vi "TC560-Write Command Data.vi"(8 "error in":errorcluster, 11 "Configuration":T1={"Connection Setting"={"VISA Resource Name"="", "Baud Rate"=9600, "Parity"=0, "Flow Control"=0}, "Wait For Read"=0} {"Connection Setting"."Flow Control" items=["None", "XON/XOFF", "RTS/CTS", "XON/XOFF & RTS/CTS", "DTR/DSR", "XON/XOFF & DTR/DSR"]; "Connection Setting"."Parity" items=["None", "Odd", "Even", "Mark", "Space"]; "Connection Setting"."Baud Rate" items=["2400"=2400, "4800"=4800, "9600"=9600]}) -> (0 "error out":errorcluster)   [LabVIEW 2018]
uses:
  Data Def/TC560-Configuration.ctl
  Data Def/TC560-Connection Setting.ctl
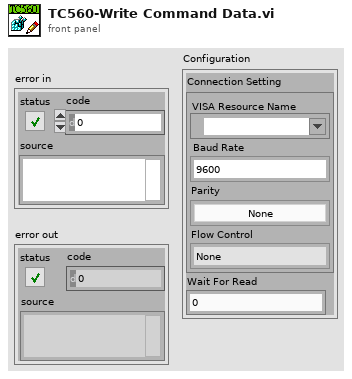
[diagram p1: front panel]
types:
  T1 = typedef "TC560-Configuration.ctl" = cluster{"Connection Setting":T2, "Wait For Read":u32}
  T2 = typedef "TC560-Connection Setting.ctl" = cluster{"VISA Resource Name":refnum<visa-resource-name>, "Baud Rate":u32, "Parity":u16, "Flow Control":u16}
  T3 = enum16{"open", "replace", "create", "open or create", "replace or create", "replace or create with confirmation"}
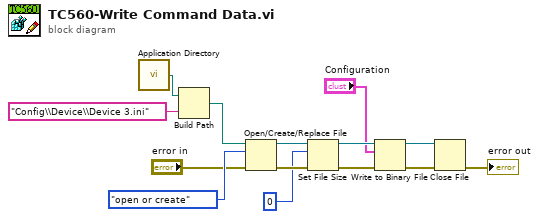
[diagram p0: block diagram]
diagram:
  n1 = call <vilib>:"Application Directory.vi"() -> ("Application Directory"=w11:path)
  n2 = Build Path(base path=w11, name or relative path="Config\\Device\\Device 3.ini") -> (appended path=w4:path)
  n3 = Open/Create/Replace File(file path (use dialog)=w4, error in="error in", operation (0:open)=T3."open or create") -> (refnum out=w8:refnum<file>, error out=w9:errorcluster)  [unwired: 3 in, 1 out]
  n4 = Set File Size(4:w9, 6:i64 0 ("size (in bytes)"), 7:w8) -> (0:w6:errorcluster, 3:w7:refnum<file>)
  n5 = Write to Binary File(file (use dialog)=w7, data="Configuration", error in=w6) -> (refnum out=w12:refnum<file>, error out=w13:errorcluster)  [unwired: 3 in, 1 out]
  n6 = Close File(refnum=w12, error in=w13) -> (error out=→"error out":errorcluster)  [unwired: 1 out]
